vi "UpdateTrendPoints.vi"(8 "error in (no error)":errorcluster, 9 "Group":T1, 10 "DataSets":T7[](array[typedef]), 11 "TrendPoints in":T5[](array[typedef])) -> (0 "error out":errorcluster, 3 "TrendPoints out":T5[](array[typedef]))   [LabVIEW 2017, in "McsaStartupAnalysis.lvlib"]
uses:
  <vilib>/addons/InsightCM/Devices/Shared/Mcsa/McsaStartupAnalysis/McsaStartupAnalysis.lvlib
  <vilib>/addons/InsightCM/Devices/Shared/Common/DataEvent/controls/DataSet.ctl
  <vilib>/addons/InsightCM/MessageBus/Base/controls/DataSetMetadata.ctl
  <vilib>/addons/InsightCM/MessageBus/Base/controls/KeyValuePair.ctl
  <vilib>/addons/InsightCM/MessageBus/Base/controls/TrendPoint.ctl
  <vilib>/addons/InsightCM/Devices/Shared/Mcsa/McsaStartupAnalysis/controls/Group.ctl
  <vilib>/addons/InsightCM/Devices/Shared/Mcsa/McsaStartupAnalysis/controls/ChannelForStartup.ctl
  <vilib>/addons/InsightCM/Devices/Shared/Mcsa/McsaStartupAnalysis/controls/StartupFeature.ctl
  <vilib>/addons/InsightCM/Devices/Shared/Mcsa/McsaStartupAnalysis/controls/MotorInfo.ctl
  <vilib>/addons/InsightCM/Devices/Shared/Common/DataEvent/DataEvent.lvlib
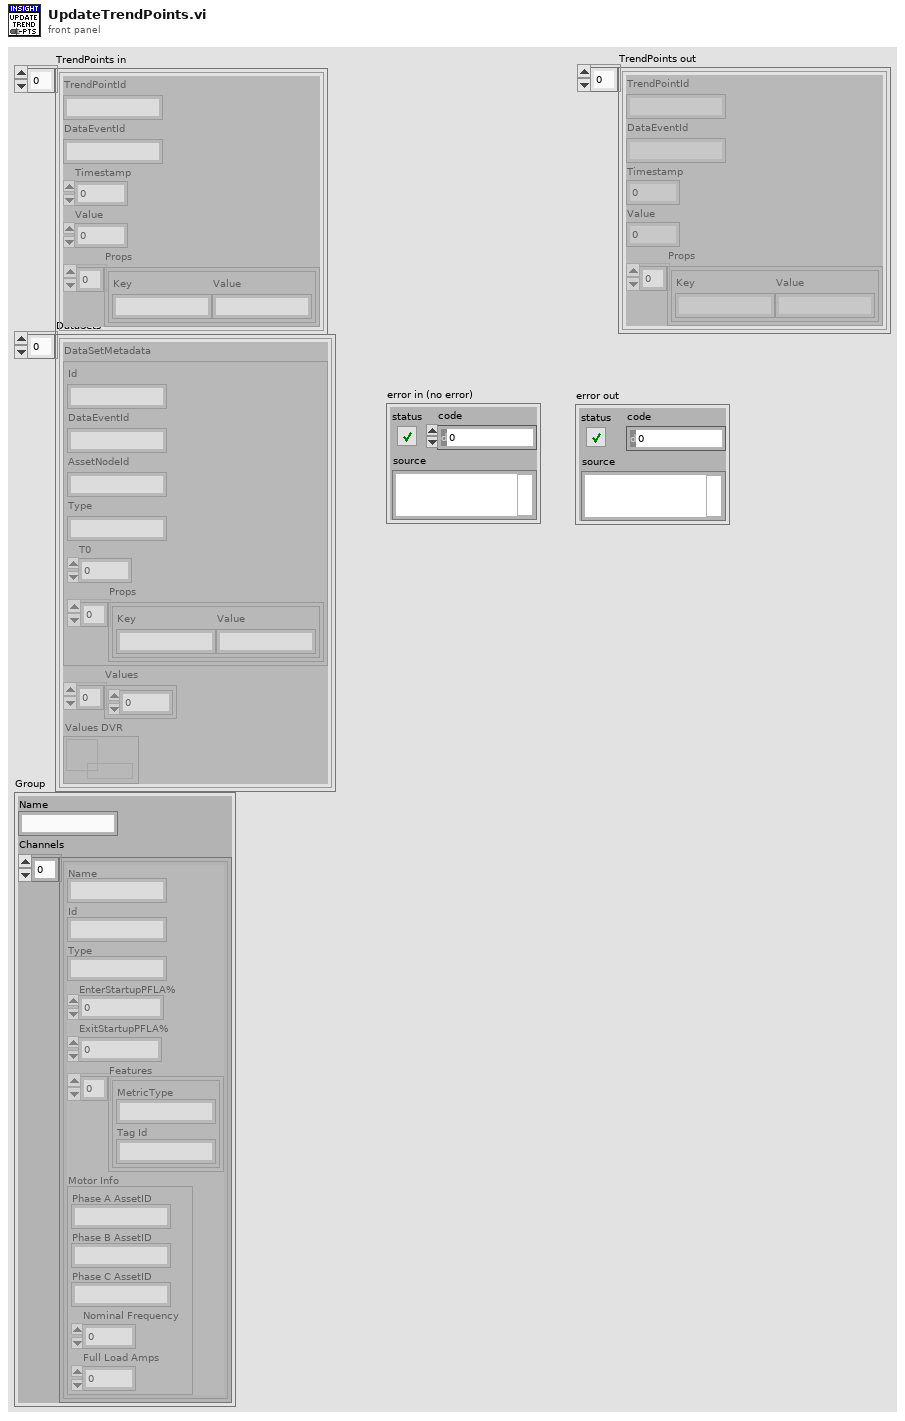
[diagram p1: front panel]
types:
  T1 = typedef "McsaStartupAnalysis.lvlib/Group.ctl" = cluster{"Name":string, "Channels":T2[]}
  T2 = typedef "McsaStartupAnalysis.lvlib/ChannelForStartup.ctl" = cluster{"Name":string, "Id":string, "Type":string, "EnterStartupPFLA%":dbl, "ExitStartupPFLA%":dbl, "Features":T3[], "Motor Info":T4}
  T3 = typedef "McsaStartupAnalysis.lvlib/StartupFeature.ctl" = cluster{"MetricType":string, "Tag Id":string}
  T4 = typedef "McsaStartupAnalysis.lvlib/MotorInfo.ctl" = cluster{"Phase A AssetID":string, "Phase B AssetID":string, "Phase C AssetID":string, "Nominal Frequency":dbl, "Full Load Amps":dbl}
  T5 = typedef "TrendPoint.ctl" = cluster{"TrendPointId":string, "DataEventId":string, "Timestamp":i64, "Value":dbl, "Props":T6[]}
  T6 = typedef "KeyValuePair.ctl" = cluster{"Key":string, "Value":string}
  T7 = typedef "DataEvent.lvlib/DataSet.ctl" = cluster{"DataSetMetadata":T8, "Values":sgl[], "Values DVR":refnum<data-value>}
  T8 = typedef "DataSetMetadata.ctl" = cluster{"Id":string, "DataEventId":string, "AssetNodeId":string, "Type":string, "T0":i64, "Props":T6[]}
  T9 = cluster{"startup time":dbl, "startup peak amps":dbl}
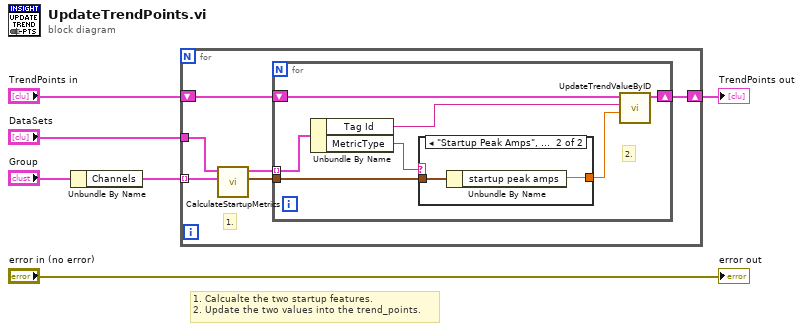
[diagram p0: block diagram]
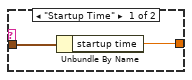
[diagram p2: hidden frame]
diagram:
  # "1. Calcualte the two startup features.\n2. Update the two values into the trend_points."
  n1 = Unbundle By Name("Group") -> ("Channels"=w3:T2[])
  n2 = for {
    tunnel: w3 -> [w8] mode=indexing
    shift-right: [w10] -> w5
    shift-left: "TrendPoints in" -> [w11]
    tunnel: "DataSets" -> [w7]
    # "1."
    n3 = call <vilib>:"CalculateStartupMetrics.vi"("Channel"=w8, "DataSets"=w7) -> ("Startup features"=w9:T9, "Features"=w12:T3[])  [unwired: 8 in]
    n4 = for {
      tunnel: w12 -> [w19] mode=indexing
      shift-right: [w16] -> w10
      shift-left: w11 -> [w18]
      tunnel: w9 -> [w14]
      # "2."
      n5 = Unbundle By Name(w19) -> ("Tag Id"=w17:string, "MetricType"=w15:string)
      n6 = case shown="\"Startup Peak Amps\", Default" w15 {
        tunnel: [w20 w22] -> w13
        tunnel: w14 -> [w21 w23]
        frame "Startup Time" {
          n7 = Unbundle By Name(w21) -> ("startup time"=w20:dbl)
        }
        frame "Startup Peak Amps", Default {
          n8 = Unbundle By Name(w23) -> ("startup peak amps"=w22:dbl)
        }
      }
      n9 = call <vilib>:"UpdateTrendValueByID.vi"("Value"=w13, "TrendPoints id"=w17, "TrendPoints in"=w18) -> ("TrendPoints out"=w16:T5[])  [unwired: 8 in]
    }
  }
  "TrendPoints out" <- w5
  "error out" <- "error in (no error)"
